vi "Shutdown Network Sink Endpoint.vi"(8 "error in (no error)":errorcluster, 11 "Network Sink Endpoint in":refnum<class "Network Sink Endpoint.lvclass">) -> (0 "error out":errorcluster)   [LabVIEW 2019, in "Network Sink.lvlib" / "Network Sink Endpoint.lvclass"]
uses:
  <vilib>/gpm_packages/@cs/event-logger/Source/Network Sink/Network Sink Endpoint/Network Sink Endpoint.lvclass
  <vilib>/gpm_packages/@cs/event-logger/Source/Network Sink/Network Sink Endpoint/Network Sink Endpoint.lvclass/Network Sink Endpoint.ctl
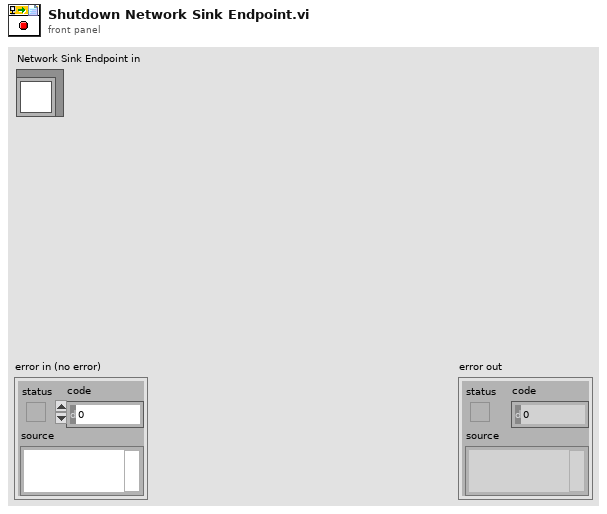
[diagram p1: front panel]
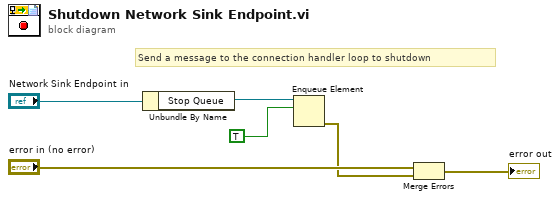
[diagram p0: block diagram]
diagram:
  # "Send a message to the connection handler loop to shutdown"
  n1 = Unbundle By Name("Network Sink Endpoint in") -> ("Stop Queue"=w5:refnum<queue>)
  n2 = Enqueue Element(queue=w5, element=TRUE) -> (error out=w2:errorcluster)  [unwired: 2 in, 2 out]
  n3 = Merge Errors("error in (no error)", w2) -> (→"error out":errorcluster)
